vi "pmu_FPGA Unlocked Seconds NIGPS.vi"(11 "locked?":bool) -> (3 "unlocked seconds (s)":u32=5)   [LabVIEW 2013]
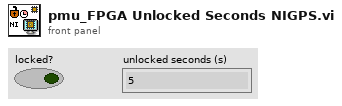
[diagram p1: front panel]
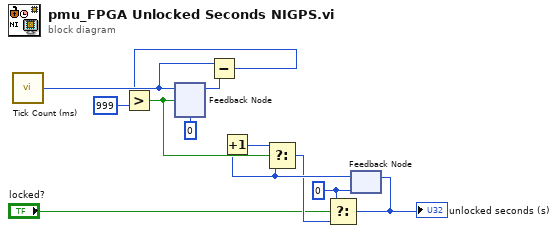
[diagram p0: block diagram]
diagram:
  w7 = u32 0 ("Unlocked Seconds")
  n1 = call "Tick Count (ms)"() -> ("Tick Count(mSec)"=w9:u32)
  n2 = feedback #1(u32 0 ("Tick Count(mSec)")) -> (w10:u32)
  n3 = Subtract(x=w9, y=w10) -> (x-y=w2:u32)
  n4 = Greater?(x=w2, y=u32 999) -> (0:w8:bool)
  n5 = feedback-in #1(w9, w8) -> ()
  n6 = feedback #2(w7) -> (w5:u32)
  n7 = Increment(x=w5) -> (x+1=w6:u32)
  n8 = Select(t=w6, s=w8, f=w5) -> (s? t:f=w4:u32)
  n9 = Select(t=w7, s="locked?", f=w4) -> (s? t:f=w3:u32)
  "unlocked seconds (s)" <- w3
  n10 = feedback-in #2(w3) -> ()
